vi "Drive Off HAB2.vi"(6 "Right Current Drawn":dbl=7.625, 7 "Left Position":dbl, 8 "Right Velocity":dbl, 9 "Right Position":dbl, 10 "Left Current Drawn":dbl=5.125, 11 "Left Velocity":dbl) -> (0 "Right Output":dbl=-0.3, 1 "Zero Encoders":bool=TRUE, 2 "Control Mode":T1 items=["PercentOutput"=0, "Position"=1, "Velocity"=2, "Current"=3, "Follower"=5, "MotionProfile"=6, "MotionMagic"=7, "MotionProfileArc"=10, "Disabled"=15], 3 "Left Output":dbl=-0.3, 4 "DONE":bool, 5 "Step":enum16{"Go Forward", "Go Backward", "Set Home"}(ring)=enum."Go Backward")   [LabVIEW 2018]
uses:
  <vilib>/Rock Robotics/WPI/ThirdParty/Phoenix-LabVIEW/Motor Controller/Controls/CTRE_Phoenix_MotorControl_ControlMode.ctl
panel:
  in  "Moving Backwards throttle":dbl=-0.3
  in  "Right MM Setpoint":dbl=4096.0
  in  "Left MM Setpoint":dbl=4096.0
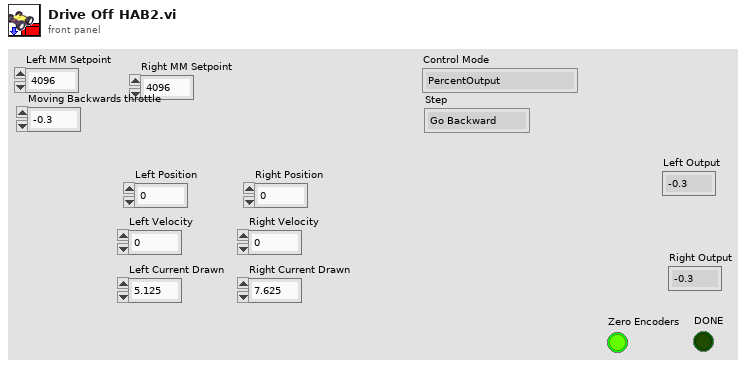
[diagram p1: front panel]
types:
  T1 = typedef "CTRE_Phoenix_MotorControl_ControlMode.ctl" = u16
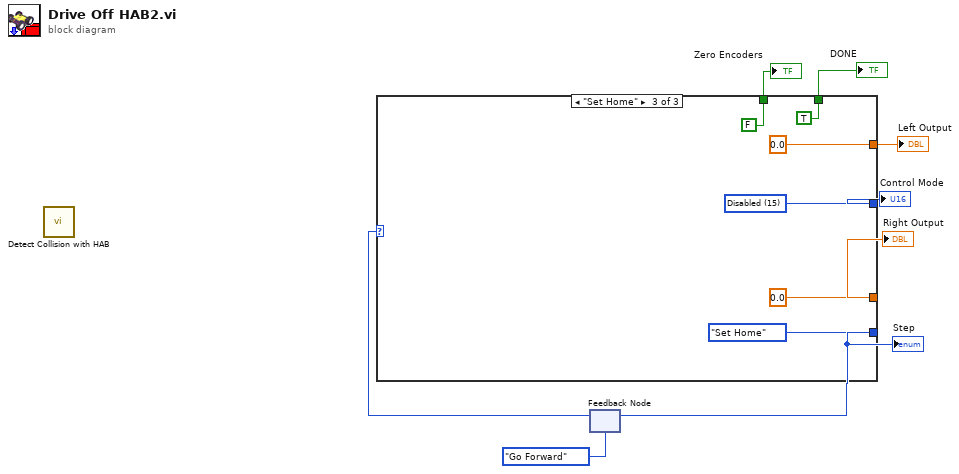
[diagram p0: block diagram]
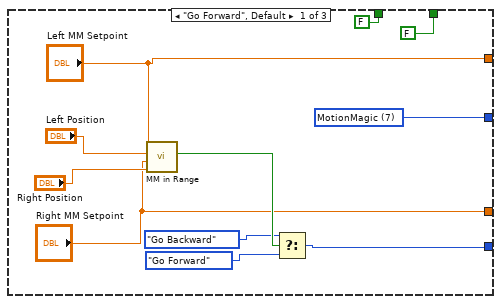
[diagram p2: hidden frame]
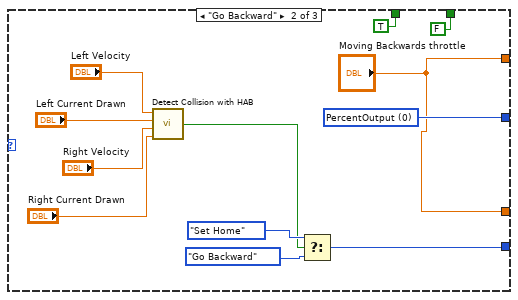
[diagram p3: hidden frame]
diagram:
  n1 = call "Detect Collision with HAB.vi"() -> ()  [unwired: 4 in, 1 out]
  n2 = feedback #1(enum16{"Go Forward", "Go Backward", "Set Home"}."Go Forward") -> (w5:enum16{"Go Forward", "Go Backward", "Set Home"})
  n3 = case shown="\"Set Home\"" w5 {
    tunnel: [w19 w31 w36] -> w8
    tunnel: ["Left MM Setpoint" "Moving Backwards throttle" 0.0 ("Left Output")] -> w7
    tunnel: ["Right MM Setpoint" "Moving Backwards throttle" 0.0 ("Right Output")] -> w6
    tunnel: [w15 w30 enum16{"Go Forward", "Go Backward", "Set Home"}."Set Home"] -> w4
    tunnel: [FALSE ("DONE/Zero Encoders") TRUE ("DONE/Zero Encoders") FALSE ("DONE/Zero Encoders")] -> w2
    tunnel: [FALSE ("DONE/Zero Encoders") FALSE ("DONE/Zero Encoders") TRUE ("DONE/Zero Encoders")] -> w1
    frame "Go Forward", Default {
      w19 = T1 7 items=["PercentOutput"=0, "Position"=1, "Velocity"=2, "Current"=3, "Follower"=5, "MotionProfile"=6, "MotionMagic"=7, "MotionProfileArc"=10, "Disabled"=15] ("Control Mode")
      n4 = call "MM in Range.vi"("Right Position"="Right Position", "Right Setpoint"="Right MM Setpoint", "Left position"="Left Position", "Left Setpoint"="Left MM Setpoint") -> ("\"Done with step\" enough"=w18:bool)  [unwired: 7 in]
      n5 = Select(t=enum16{"Go Forward", "Go Backward", "Set Home"}."Go Backward", s=w18, f=enum16{"Go Forward", "Go Backward", "Set Home"}."Go Forward") -> (s? t:f=w15:enum16{"Go Forward", "Go Backward", "Set Home"})
    }
    frame "Go Backward" {
      w31 = T1 0 items=["PercentOutput"=0, "Position"=1, "Velocity"=2, "Current"=3, "Follower"=5, "MotionProfile"=6, "MotionMagic"=7, "MotionProfileArc"=10, "Disabled"=15] ("Control Mode")
      n6 = call "Detect Collision with HAB.vi"("Right Current"="Right Current Drawn", "Right Velocity"="Right Velocity", "Left Current"="Left Current Drawn", "Left Velocity"="Left Velocity") -> ("HIT WALL"=w27:bool)
      n7 = Select(t=enum16{"Go Forward", "Go Backward", "Set Home"}."Set Home", s=w27, f=enum16{"Go Forward", "Go Backward", "Set Home"}."Go Backward") -> (s? t:f=w30:enum16{"Go Forward", "Go Backward", "Set Home"})
    }
    frame "Set Home" {
      w36 = T1 15 items=["PercentOutput"=0, "Position"=1, "Velocity"=2, "Current"=3, "Follower"=5, "MotionProfile"=6, "MotionMagic"=7, "MotionProfileArc"=10, "Disabled"=15] ("Control Mode")
    }
  }
  "Left Output" <- w7
  "Right Output" <- w6
  "Control Mode" <- w8
  "Zero Encoders" <- w2
  "Step" <- w4
  "DONE" <- w1
  n8 = feedback-in #1(w4) -> ()
